vi "Formula_Node_Ejercicio.vi"() -> ()   [LabVIEW 2020]
panel:
  out "XY Graph":cluster{dbl[], dbl[]}(graph)
  out "Waveform Graph":dbl[](graph)
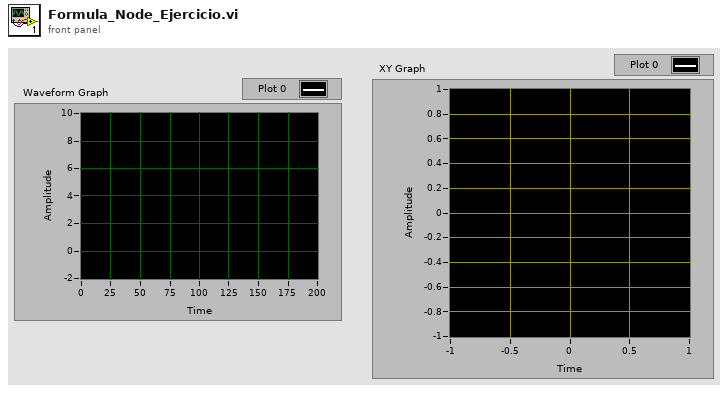
[diagram p1: front panel]
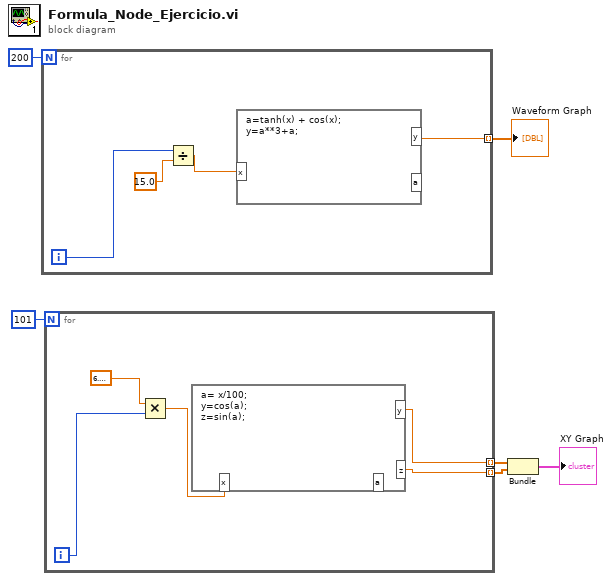
[diagram p0: block diagram]
diagram:
  n1 = for {
    N: 200 -> [_]
    tunnel: [w8] -> w5 mode=indexing
    i -> [w9]
    n2 = Divide(x=w9, y=15.0) -> (x/y=w7:dbl)
    n3 = formula code="a=tanh(x) + cos(x);\ny=a**3+a;"("x"=w7) -> ("y"=w8:dbl)  [unwired: 1 out]
  }
  "Waveform Graph" <- w5
  n4 = for {
    N: 101 -> [_]
    tunnel: [w12] -> w3 mode=indexing
    tunnel: [w11] -> w2 mode=indexing
    i -> [w15]
    n5 = Multiply(x=6.283185307179586, y=w15) -> (x*y=w13:dbl)
    n6 = formula code="a= x/100;\ny=cos(a);\nz=sin(a);"("x"=w13) -> ("y"=w12:dbl, "z"=w11:dbl)  [unwired: 1 out]
  }
  n7 = Bundle(w3, w2) -> (→"XY Graph":cluster{dbl[], dbl[]})  [unwired: 1 in]
